vi "Init.vi"(8 "error in (no error)":errorcluster, 10 "Config Query":refnum<class "CConfig Query.lvclass">) -> (0 "error out":errorcluster, 3 "Step In Query out":refnum<class "Step In Query.lvclass">)   [LabVIEW 2013, in "Step In Query.lvclass"]
doc: "Copyright 2018, Carya Automatisering, Wiebe Walstra."
uses:
  Step In Query.lvclass
  CConfig Query.lvclass
  Step In Query.lvclass/Step In Query.ctl
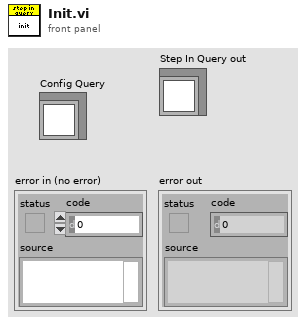
[diagram p1: front panel]
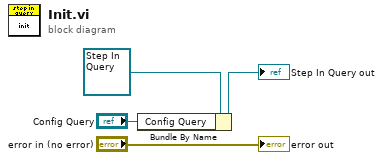
[diagram p0: block diagram]
diagram:
  n1 = Bundle By Name(cluster=refnum<class "Step In Query.lvclass"> refnum ("Step In Query in"), "Config Query"="Config Query") -> (→"Step In Query out":refnum<class "Step In Query.lvclass">)
  "error out" <- "error in (no error)"
